vi "TurnOffDivideByFiceClockingHiSpeedDevice.vi"(2 "error in (no error)":errorcluster, 3 "handle":u32) -> (0 "error out":errorcluster, 1 "result":u32)   [LabVIEW 2010]
uses:
  FTCSPI.dll
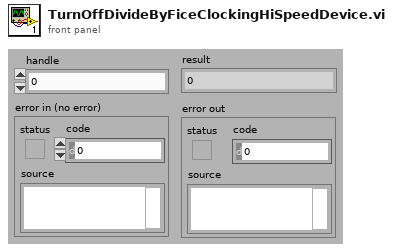
[diagram p1: front panel]
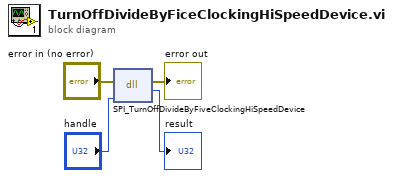
[diagram p0: block diagram]
diagram:
  n1 = dll-call lib="C:/Users/Administrator/Documents/GitHub/labview/FPGA/FTCSPI.dll" fn="SPI_TurnOffDivideByFiveClockingHiSpeedDevice"(error in="error in (no error)", "handle"="handle") -> (error out=→"error out":errorcluster, "result"=→"result":u32)  [unwired: 3 in, 1 out]
